vi "openImaFile.vi"(8 "error in (no error)":errorcluster, 9 "nbrCol":i32, 10 "nbrLine":i32, 11 "Logging Configuration":T1 {"NbrIma" min=1 step=1}) -> (0 "error out":errorcluster)   [LabVIEW 2020, in "Logging.lvlib"]
uses:
  LOGGING/Logging.lvlib
  LOGGING/Logging Configuration.ctl
  BigDataFits.ctl
  DataTyp_Header.ctl
  ClustBigFilFits.ctl
panel:
  in  "name":string="ima"
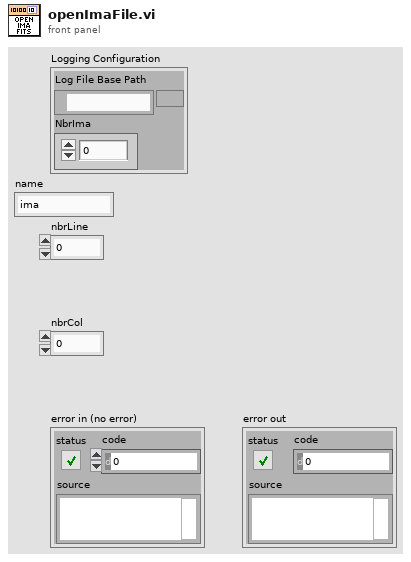
[diagram p1: front panel]
types:
  T1 = typedef "Logging.lvlib/Logging Configuration.ctl" = cluster{"Log File Base Path":path, "NbrIma":i32}
  T2 = typedef "ClustBigFilFits.ctl" = cluster{"file (use dialog)":path, "Type de données":T3, "Commentaire":string, "naxis1":i32, "naxis2":i32, "naxis3":i32, "Exptime":sgl}
  T3 = typedef "DataTyp_Header.ctl" = enum16{"U8 (unsigned integer 8bit)", "I16 (signed integer 16bit)", "U16 (unsigned integer 16 bit)", "I32 (signed integer 32bit)", "U32 (unsigned integer 32 bit)", "SGL (float 32bit)", "DBL(float 64bit)", "complex (2xfloat 64bit)"}
  T4 = typedef "BigDataFits.ctl" = enum16{"Init", "WritHeader", "WritData", "Close"}
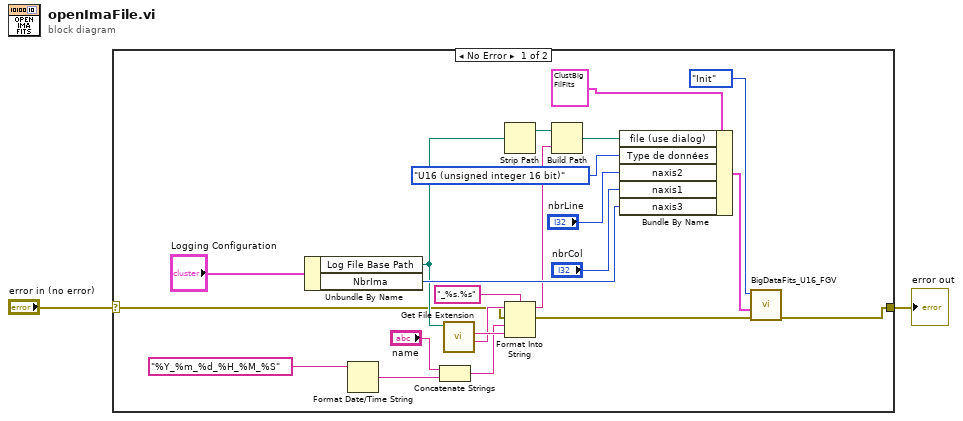
[diagram p0: block diagram]
diagram:
  n1 = case shown="No Error" "error in (no error)" {
    selector: "error in (no error)" -> [w4 w25]
    tunnel: [w16 w25] -> w2
    frame No Error {
      n2 = Unbundle By Name("Logging Configuration") -> ("Log File Base Path"=w7:path, "NbrIma"=w21:i32)
      n3 = Format Date/Time String(time format string (%c)="%Y_%m_%d_%H_%M_%S") -> (date/time string=w12:string)  [unwired: 2 in]
      n4 = Concatenate Strings("name", w12) -> (w6:string)
      n5 = call <vilib>:"Get File Extension.vi"("file"=w7) -> ("filename without extension"=w9:string, "lowercase file extension"=w13:string)  [unwired: 6 in, 3 out]
      n6 = Strip Path(path=w7) -> (stripped path=w10:path)  [unwired: 1 out]
      n7 = Format Into String(format string="_%s.%s", initial string=w9, error in=w4, w6, w13) -> (resulting string=w14:string, error out=w3:errorcluster)
      n8 = Build Path(base path=w10, name or relative path=w14) -> (appended path=w20:path)
      n9 = Bundle By Name(cluster=T2 {"file (use dialog)"=path "D:/DATA/Imatest.fits", "Type de données"=enum."U16 (unsigned integer 16 bit)", "Commentaire"="", "naxis1"=0, "naxis2"=0, "naxis3"=1, "Exptime"=1.0} ("ClustBigFilFits"), "file (use dialog)"=w20, "Type de données"=DataTyp_Header."U16 (unsigned integer 16 bit)", "naxis2"="nbrLine", "naxis1"="nbrCol", "naxis3"=w21) -> (w18:T2)
      n10 = call "BigDataFits_U16_FGV.vi"("InError"=w3, "ClustBigFilFits"=w18, "Énum"=BigDataFits."Init") -> ("sortie d'erreur"=w16:errorcluster)  [unwired: 8 in]
    }
    frame Error {
    }
  }
  "error out" <- w2
